vi "allUkuleleFreq.vi"() -> (3 "array of frequencies":dbl[](array[numeric]))   [LabVIEW 2019]
panel:
  in  "Numeric":dbl
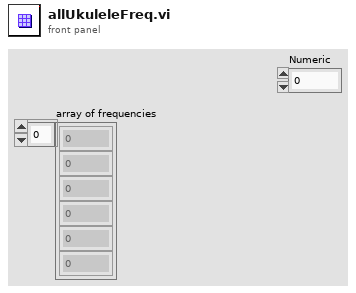
[diagram p1: front panel]
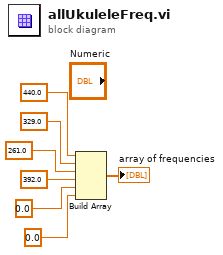
[diagram p0: block diagram]
diagram:
  n1 = Build Array(440.0 ("element"), 329.0 ("element"), 261.0 ("element"), 392.0 ("element"), 0.0 ("element"), 0.0 ("element")) -> (→"array of frequencies":dbl[])
